vi "maximize field component.vi"() -> ()   [LabVIEW 2013]
uses:
  gaussmeter/gaussmeter channels.ctl
  config.vi
panel:
  in  "start angle":dbl
  out "error out":errorcluster
  in  "error in (no error)":errorcluster
  in  "vector field component":T1
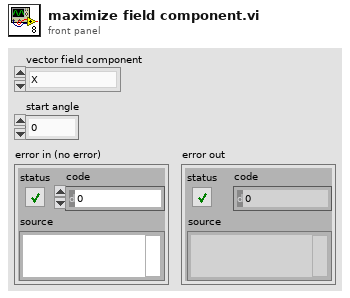
[diagram p1: front panel]
types:
  T1 = typedef "gaussmeter channels.ctl" = enum16{"X", "Y", "Z", "Vec"}
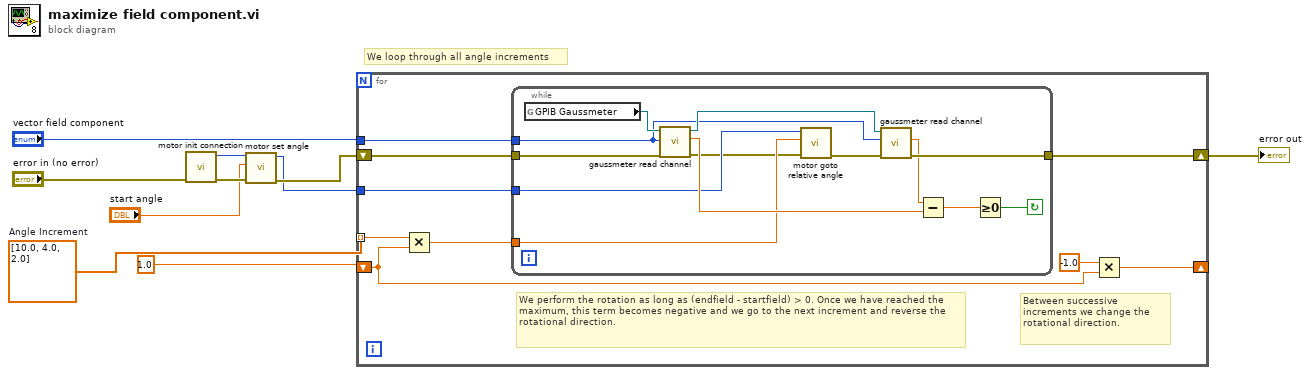
[diagram p0: block diagram]
diagram:
  w10 = dbl[] [10.0, 4.0, 2.0]  # Angle Increment
  # "We loop through all angle increments"
  n1 = call "motor init connection.vi"("error in (no error)"="error in (no error)") -> ("error out"=w4:errorcluster, "Handle Out"=w5:i32)  [unwired: 9 in]
  n2 = call "motor set angle.vi"("error in (no error)"=w4, "angle"="start angle", "Handle In"=w5) -> ("error out"=w3:errorcluster, "Handle Out"=w2:i32)  [unwired: 7 in]
  n3 = for {
    tunnel: w10 -> [w18] mode=indexing
    tunnel: "vector field component" -> [w19]
    shift-right: [w16] -> _
    shift-left: 1.0 -> [w15]
    shift-right: [w13] -> w7
    shift-left: w3 -> [w12]
    tunnel: w2 -> [w11]
    # "We perform the rotation as long as (endfield - startfield) > 0. Once we have reached the maximum, this term becomes negative and we go to the next increment and reverse the rotational direction."
    # "Between successive increments we change the rotational direction."
    n4 = Multiply(x=w18, y=w15) -> (x*y=w17:dbl)
    n5 = while {
      tunnel: w12 -> [w31]
      tunnel: w19 -> [w25]
      tunnel: w17 -> [w22]
      tunnel: [w28] -> w13
      tunnel: w11 -> [w21]
      stop <- w29 continue-if-true
      n6 = global read "config.vi" "GPIB Gaussmeter"() -> (w32:refnum<visa-resource-name>)
      n7 = call "gaussmeter read channel.vi"("error in (no error)"=w31, "channel"=w25, "VISA resource name"=w32) -> ("error out"=w20:errorcluster, "magnetic field (T)"=w26:dbl, "VISA resource name 2"=w30:refnum<visa-resource-name>)  [unwired: 6 in]
      n8 = call "motor goto relative angle.vi"("error in (no error)"=w20, "angle"=w22, "Handle In"=w21) -> ("error out"=w23:errorcluster)  [unwired: 7 in, 1 out]
      n9 = call "gaussmeter read channel.vi"("error in (no error)"=w23, "channel"=w25, "VISA resource name"=w30) -> ("error out"=w28:errorcluster, "magnetic field (T)"=w27:dbl)  [unwired: 6 in, 1 out]
      n10 = Subtract(x=w27, y=w26) -> (x-y=w24:dbl)
      n11 = Greater Or Equal To 0?(x=w24) -> (x >= 0?=w29:bool)
    }
    n12 = Multiply(x=-1.0, y=w15) -> (x*y=w16:dbl)
  }
  "error out" <- w7
